vi "SetupGenerator.vi"(5 "Freq (Hz)":dbl=1250000000.0 format="%#_6p", 6 "DAC Codes":u16[](array[numeric]), 7 "NumSamples":u32=1024, 8 "error in":errorcluster, 9 "Delay bw waves [cycles]":u32, 10 "Waves Per Pixel":i16=1, 11 "RIO Device IN":T1="RIO0" caption="RIO Device") -> (0 "error out":errorcluster)   [LabVIEW 2018]
uses:
  <vilib>/userdefined/High Color/nirio_resource_hc.ctl
  <vilib>/FPGAPlugInAG/Dynamic/niLvFpga_Close_Dynamic.vi
  <vilib>/Utility/error.llb/Error Cluster From Error Code.vi
  <vilib>/rvi/errors/niLvFpgaAdjustHostInterfaceError.vi
  <vilib>/rvi/interface/nirviCloseFPGA/nirviCloseFPGA.xnode
  <vilib>/rvi/interface/nirviReadWriteControl/nirviReadWriteControl.xnode
  <vilib>/rvi/interface/Simulation/niFpgaSimulationCallBeginRW.vi
  NiFpgaLv.dll
panel:
  in  "FPGA 1212 VI Reference":refnum<k20>
  out "Waveform Graph":u16[](graph)
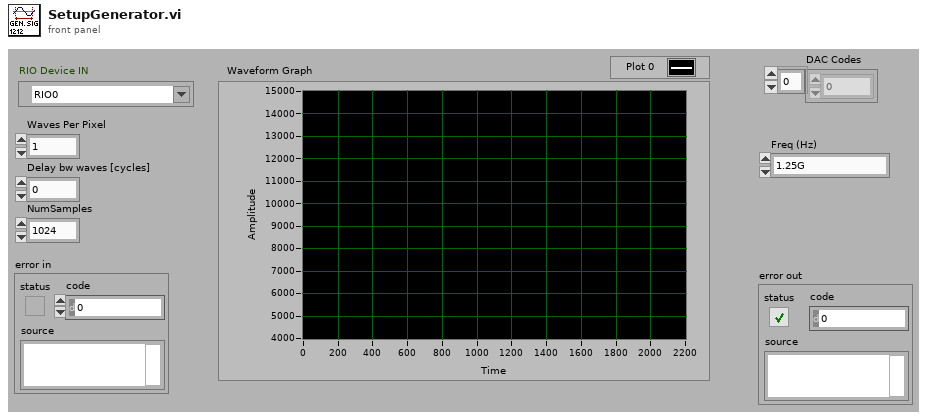
[diagram p1: front panel]
types:
  T1 = typedef "nirio_resource_hc.ctl" = tag
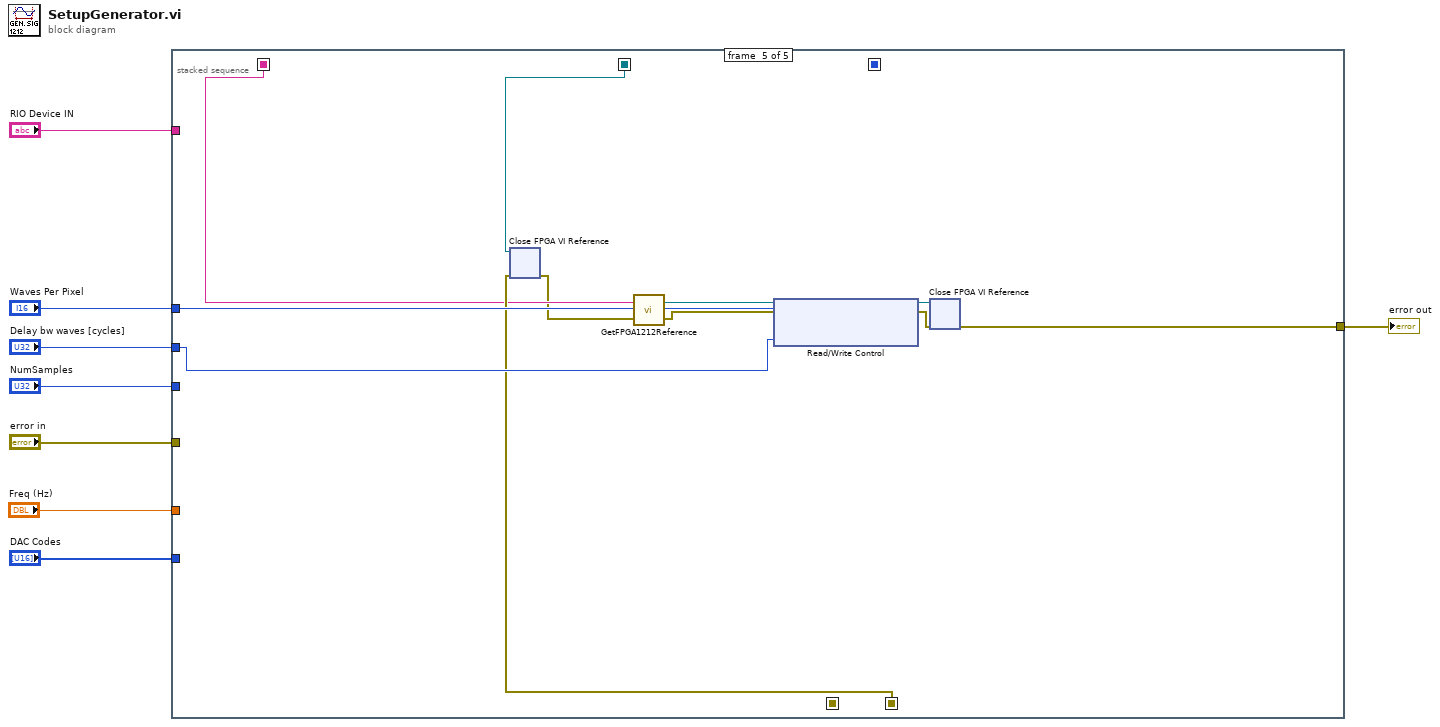
[diagram p0: block diagram]
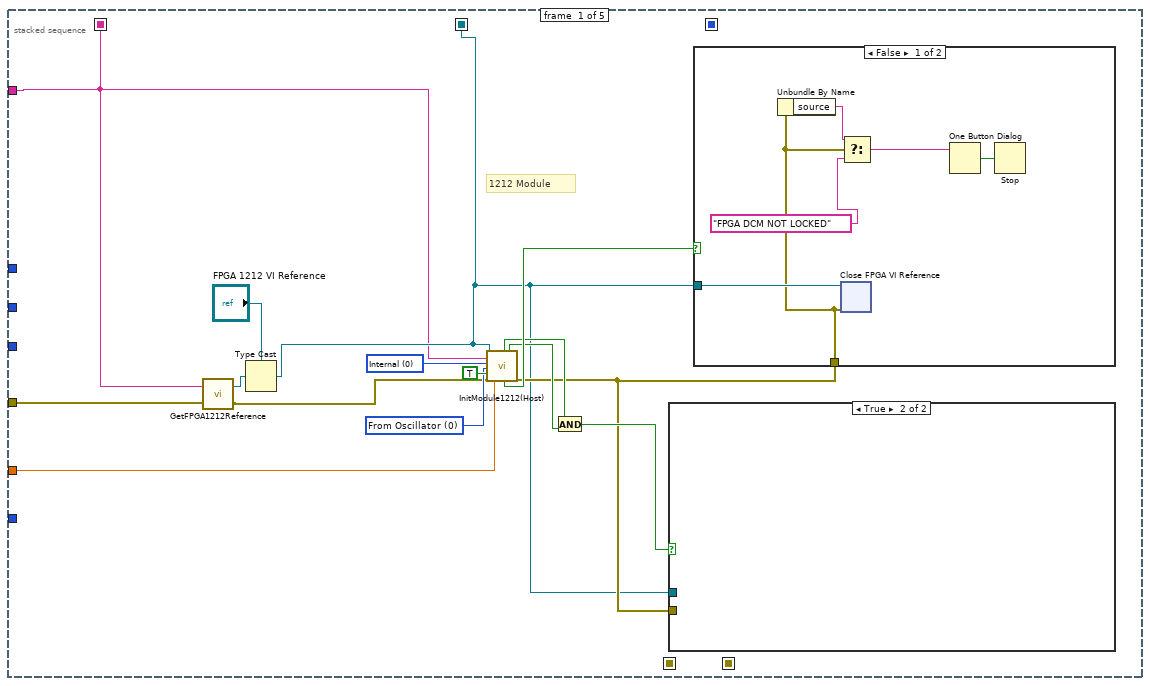
[diagram p2: hidden frame]
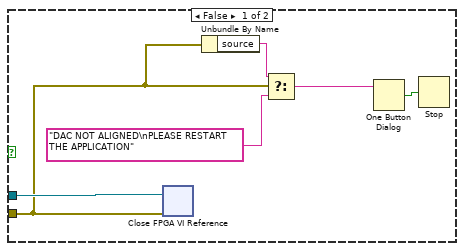
[diagram p3: hidden frame]
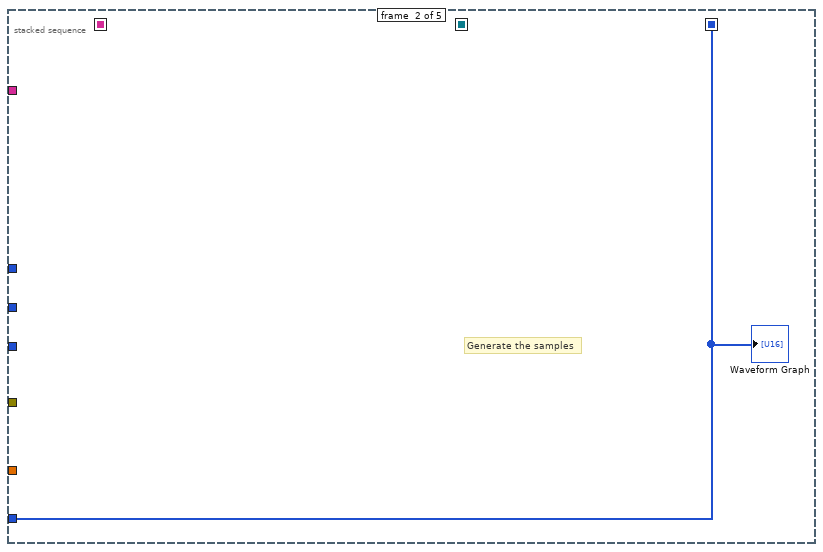
[diagram p5: hidden frame]
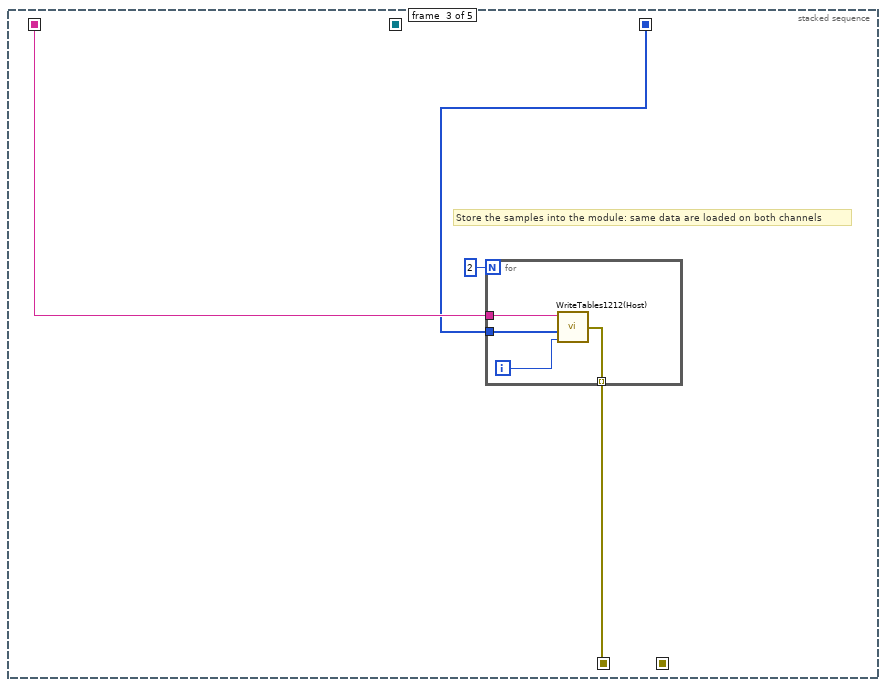
[diagram p6: hidden frame]
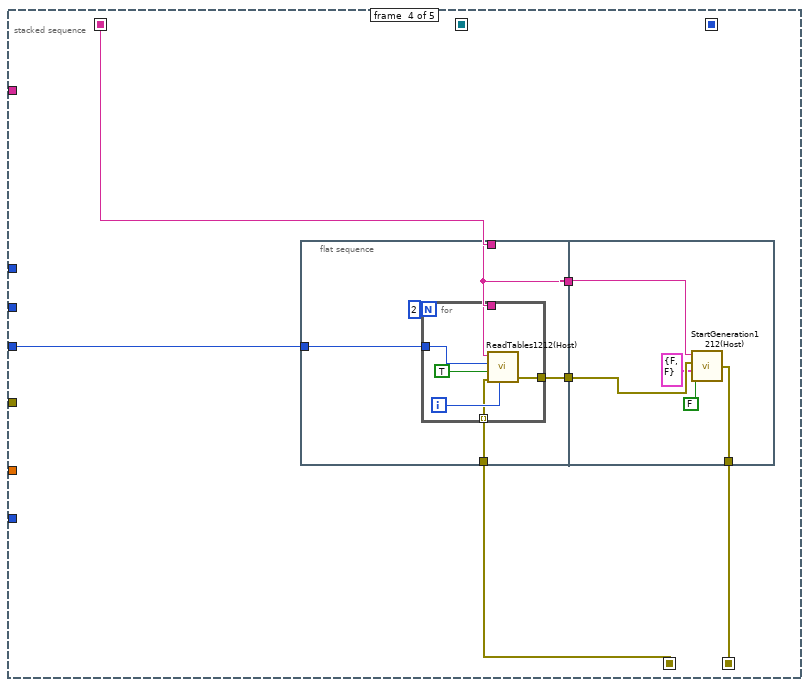
[diagram p7: hidden frame]
diagram:
  n1 = stacked-sequence {
    seq-local: [w11 _ _ _ _] -> [_ _ w39 w48 w70]
    seq-local: [_ w36 _ _ _] -> [_ _ w38 _ _]
    seq-local: [w13 _ _ _ _] -> [_ _ _ _ w77]
    seq-local: [_ _ w37 _ _] -> [_ _ _ w46 _]
    seq-local: [_ _ _ w45 _] -> [_ _ _ _ w71]
    tunnel: "RIO Device IN" -> [w11 _ _ _ _]
    tunnel: "error in" -> [w10 _ _ _ _]
    tunnel: "DAC Codes" -> [_ w36 _ _ _]
    tunnel: "NumSamples" -> [_ _ _ w47 _]
    tunnel: "Waves Per Pixel" -> [_ _ _ _ w76]
    tunnel: "Delay bw waves [cycles]" -> [_ _ _ _ w75]
    tunnel: [_ _ _ _ w72] -> w3
    tunnel: "Freq (Hz)" -> [w9 _ _ _ _]
    frame #0 {
      w16 = u8 0 items=["From Oscillator", "From FPGA Clock"] ("INTERNAL CLOCK")
      w17 = u8 0 items=["Internal", "External (From SMA)"] ("CLOCK SELECTION")
      # "1212 Module"
      n2 = call "GetFPGA1212Reference.vi"("error in"=w10, "RIO Device IN"=w11) -> ("error out"=w15:errorcluster, "FPGA VI Reference Out"=w14:refnum<k20>)
      n3 = Type Cast(type="FPGA 1212 VI Reference", x=w14) -> (*(type *) &x=w13:refnum<k20>)
      n4 = call "InitModule1212(Host).vi"("FPGA 1212 VI Reference"=w13, "RIO Device IN"=w11, "CLOCK SELECTION"=w17, "INTERNAL CLOCK"=w16, "Master"=TRUE, "error in"=w15, "Freq (Hz)"=w9) -> ("DAC A Aligned"=w21:bool, "FPGA DCM LOCKED"=w23:bool, "DAC B Aligned"=w20:bool, "error out"=w19:errorcluster)  [unwired: 6 in, 3 out]
      n5 = And(x=w21, y=w20) -> (x .and. y?=w22:bool)
      n6 = case shown="True" w22 {
        tunnel: w13 -> [w29 _]
        tunnel: w19 -> [w24 _]
        frame False {
          n7 = xnode "Close FPGA VI Reference"("FPGA VI Reference In"=w29, "error in"=w24) -> ()  [unwired: 1 out]
          n8 = Unbundle By Name(w24) -> ("source"=w25:string)
          n9 = Select(t=w25, s=w24, f="DAC NOT ALIGNED\nPLEASE RESTART THE APPLICATION" ("message")) -> (s? t:f=w26:string)
          n10 = One Button Dialog(message=w26) -> (true=w27:bool)  [unwired: 1 in]
          n11 = Stop(stop? (T)=w27) -> ()
        }
        frame True {
        }
      }
      n12 = case shown="False" w23 {
        tunnel: w13 -> [w34 _]
        tunnel: w19 -> [w31 _]
        frame False {
          n13 = Unbundle By Name(w31) -> ("source"=w30:string)
          n14 = xnode "Close FPGA VI Reference"("FPGA VI Reference In"=w34, "error in"=w31) -> ()  [unwired: 1 out]
          n15 = Select(t=w30, s=w31, f="FPGA DCM NOT LOCKED" ("message")) -> (s? t:f=w33:string)
          n16 = One Button Dialog(message=w33) -> (true=w35:bool)  [unwired: 1 in]
          n17 = Stop(stop? (T)=w35) -> ()
        }
        frame True {
        }
      }
    }
    frame #1 {
      # "Generate the samples"
      "Waveform Graph" <- w36
    }
    frame #2 {
      # "Store the samples into the module: same data are loaded on both channels"
      n18 = for {
        N: 2 -> [_]
        tunnel: w38 -> [w44]
        tunnel: w39 -> [w42]
        tunnel: [w41] -> w37 mode=indexing
        i -> [w43]
        n19 = call "WriteTables1212(Host).vi"("Select Channel"=w43, "WavefArray"=w44, "resource name"=w42) -> ("error out"=w41:errorcluster)  [unwired: 1 in]
      }
    }
    frame #3 {
      n20 = flat-sequence {
        tunnel: [w55] -> w50
        tunnel: w48 -> [w53]
        tunnel: [w53] -> w49
        tunnel: w47 -> [w52]
        tunnel: w46 -> [w51]
        tunnel: w50 -> [w66]
        tunnel: w49 -> [w65]
        tunnel: [w62] -> w45
        frame #0 {
          n21 = for {
            N: 2 -> [_]
            tunnel: [w61] -> w55
            tunnel: w53 -> [w58]
            tunnel: w52 -> [w57]
            tunnel: w51 -> [w56] mode=indexing
            i -> [w59]
            n22 = call "ReadTables1212(Host).vi"("resource name"=w58, "NumSamples"=w57, "DDS/ARB"=TRUE, "Select Channel"=w59, "error in"=w56) -> ("error out"=w61:errorcluster)  [unwired: 3 in]
          }
        }
        frame #1 {
          n23 = call "StartGeneration1212(Host).vi"("SYNC"=FALSE, "Channel Cluster"=cluster{"CH1 ON ":bool, "CH2 ON":bool} {"CH1 ON "=FALSE, "CH2 ON"=FALSE}, "error in"=w66, "resource name"=w65) -> ("error out"=w62:errorcluster)
        }
      }
    }
    frame #4 {
      n24 = xnode "Close FPGA VI Reference"("FPGA VI Reference In"=w77, "error in"=w71) -> ("error out"=w69:errorcluster)
      n25 = call "GetFPGA1212Reference.vi"("error in"=w69, "RIO Device IN"=w70) -> ("error out"=w67:errorcluster, "FPGA VI Reference Out"=w68:refnum<k20>)
      n26 = xnode "Read/Write Control"("FPGA VI Reference In"=w68, "error in"=w67, "Waves Per Pixel"=w76, "Delay bw waves [cycles]"=w75) -> ("FPGA VI Reference Out"=w74:refnum<k20>, "error out"=w73:errorcluster)
      n27 = xnode "Close FPGA VI Reference"("FPGA VI Reference In"=w74, "error in"=w73) -> ("error out"=w72:errorcluster)
    }
  }
  "error out" <- w3
